vi "Destroy.vi"(8 "Error In":errorcluster, 11 "Compiler":refnum<class "Compiler.lvclass">) -> (0 "Error Out":errorcluster)   [LabVIEW 2017, in "Mustache.lvlib" / "Compiler.lvclass"]
uses:
  Compiler.lvclass
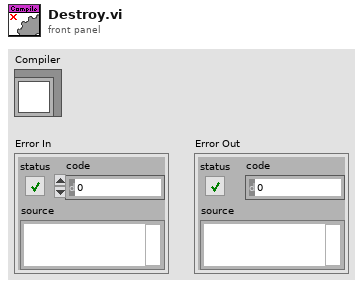
[diagram p1: front panel]
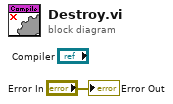
[diagram p0: block diagram]
diagram:
  "Error Out" <- "Error In"
